vi "Problem1.8.vi"() -> ()   [LabVIEW 2018]
panel:
  out "Uniform Deviate":dbl
  out "Original Random Number":dbl
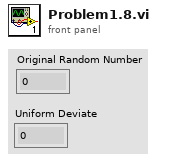
[diagram p1: front panel]
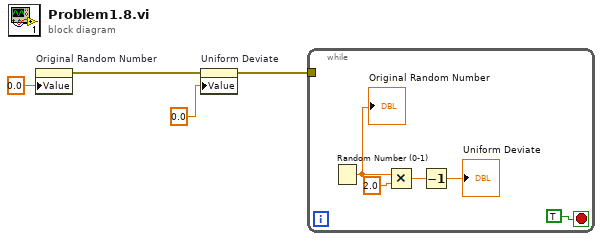
[diagram p0: block diagram]
diagram:
  n1 = property on="Original Random Number" class="DigNum (strict)"("Value"=0.0 ("Original Random Number")) -> (error out=w3:errorcluster)  [unwired: 2 in, 1 out]
  n2 = property on="Uniform Deviate" class="DigNum (strict)"(error in=w3, "Value"=0.0 ("Uniform Deviate")) -> (error out=w1:errorcluster)  [unwired: 1 in, 1 out]
  n3 = while {
    tunnel: w1 -> [_]
    stop <- TRUE stop-if-true
    n4 = Random Number (0-1)() -> (number: 0 to 1=w8:dbl)
    "Original Random Number" <- w8
    n5 = Multiply(x=w8, y=2.0) -> (x*y=w6:dbl)
    n6 = Decrement(x=w6) -> (x-1=→"Uniform Deviate":dbl)
  }
